vi "Op-List-Marker.vi"(5 "value":dbl format="%^.4e", 6 "where (min:0)":u16(ring) items=["minimum", "maximum", "at value"], 7 "variable name":string, 8 "error in (no error)":errorcluster, 9 "index":i32=1, 10 "marker function":i32(slide) max=6 scale=0.0..4.0, 11 "VISA resource name":refnum<visa-resource-name>) -> (0 "error out":errorcluster, 3 "VISA resource name out":refnum<visa-resource-name>)   [LabVIEW 2016, in "Agilent 415X Series.lvlib"]
doc: "This VI controls the marker for LIST display. Executing this VI automatically switches the display mode to LIST."
uses:
  Agilent 415X Series.lvlib
panel:
  # "This VI will change the display mode to LIST"
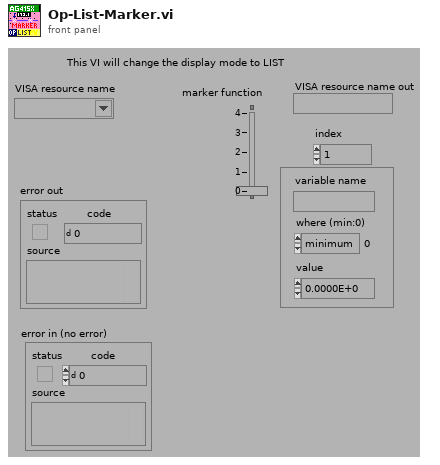
[diagram p1: front panel]
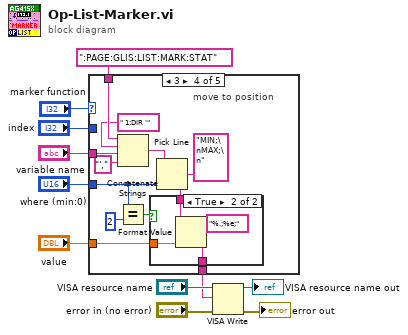
[diagram p0: block diagram]
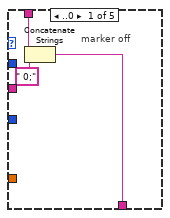
[diagram p2: hidden frame]
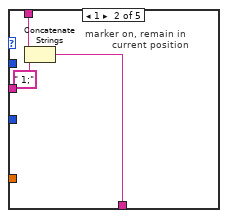
[diagram p3: hidden frame]
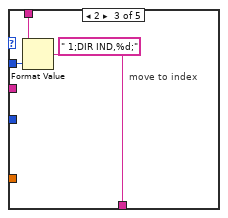
[diagram p4: hidden frame]
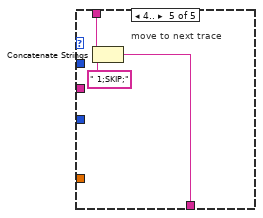
[diagram p6: hidden frame]
diagram:
  n1 = case shown="3" "marker function" {
    tunnel: ":PAGE:GLIS:LIST:MARK:STAT" -> [w14 w17 w20 w33 w41]
    tunnel: [w12 w15 w18 w26 w39] -> w6
    tunnel: "where (min:0)" -> [_ _ _ w24 _]
    tunnel: "variable name" -> [_ _ _ w31 _]
    tunnel: "index" -> [_ _ w21 _ _]
    tunnel: "value" -> [_ _ _ w25 _]
    frame ..0 {
      # "marker off"
      n2 = Concatenate Strings(w14, " 0;") -> (w12:string)
    }
    frame 1 {
      # "marker on, remain in\n         current position"
      n3 = Concatenate Strings(w17, " 1;") -> (w15:string)
    }
    frame 2 {
      # "move to index"
      n4 = Format Value(string ("")=w20, format string=" 1;DIR IND,%d;", value (0)=w21) -> (output string=w18:string)
    }
    frame 3 {
      # "move to position"
      n5 = Concatenate Strings(w33, " 1;DIR '", w31, "',") -> (w29:string)
      n6 = Equal?(x=w24, y=2) -> (x = y?=w22:bool)
      n7 = Pick Line(string ("")=w29, multi-line string="MIN;\nMAX;\n", line index=w24) -> (output string=w27:string)
      n8 = case shown="True" w22 {
        tunnel: w27 -> [w34 w38]
        tunnel: [w34 w37] -> w26
        tunnel: w25 -> [_ w36]
        frame False {
        }
        frame True {
          n9 = Format Value(string ("")=w38, format string="%.;%e;", value (0)=w36) -> (output string=w37:string)
        }
      }
    }
    frame 4.. {
      # "move to next trace"
      n10 = Concatenate Strings(w41, " 1;SKIP;") -> (w39:string)
    }
  }
  n11 = VISA Write(VISA resource name="VISA resource name", write buffer=w6, error in (no error)="error in (no error)") -> (VISA resource name out=→"VISA resource name out":refnum<visa-resource-name>, error out=→"error out":errorcluster)  [unwired: 1 out]
